vi "BuildDeleteQuery.vi"(8 "error in (no error)":errorcluster, 10 "QueryBuilderData":T1) -> (0 "error out":errorcluster, 2 "Query":string)   [LabVIEW 2022 SP3]
uses:
  DataTypes/QuiryBuilderData--Cluster.ctl
  <vilib>/Utility/error.llb/Trim Whitespace One-Sided.vi
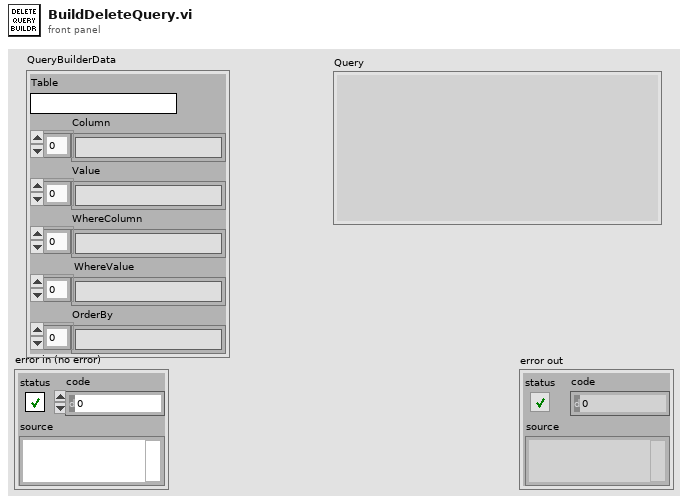
[diagram p1: front panel]
types:
  T1 = typedef "QuiryBuilderData--Cluster.ctl" = cluster{"Table":string, "Column":string[], "Value":string[], "WhereColumn":string[], "WhereValue":string[], "OrderBy":string[]}
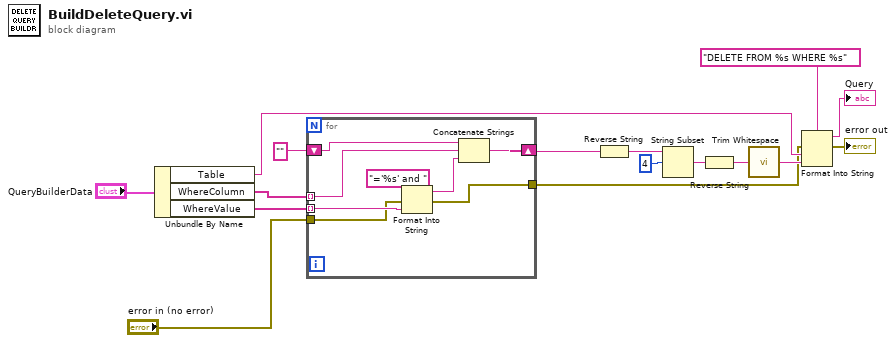
[diagram p0: block diagram]
diagram:
  n1 = Unbundle By Name("QueryBuilderData") -> ("Table"=w4:string, "WhereColumn"=w7:string[], "WhereValue"=w8:string[])
  n2 = for {
    tunnel: w7 -> [w24] mode=indexing
    shift-right: [w23] -> w15
    shift-left: "" -> [w22]
    tunnel: w8 -> [w19] mode=indexing
    tunnel: "error in (no error)" -> [w18]
    tunnel: [w17] -> w1
    n3 = Format Into String(format string="='%s' and " ("string"), error in=w18, w19) -> (resulting string=w20:string, error out=w17:errorcluster)  [unwired: 1 in]
    n4 = Concatenate Strings(w22, w24, w20) -> (w23:string)
  }
  n5 = Reverse String(1:w15) -> (0:w13:string)
  n6 = String Subset(string=w13, offset (0)=4) -> (substring=w12:string)  [unwired: 1 in]
  n7 = Reverse String(1:w12) -> (0:w11:string)
  n8 = call <vilib>:"Trim Whitespace.vi"("string"=w11) -> ("trimmed string"=w5:string)  [unwired: 1 in]
  n9 = Format Into String(format string="DELETE FROM %s WHERE %s", error in=w1, w4, w5) -> (resulting string=→"Query":string, error out=→"error out":errorcluster)  [unwired: 1 in]
